vi "Replace Outside Typedef Const.vi"(8 "error in":errorcluster, 10 "non-library vi[]":string[](array[string]), 11 "target directory":path) -> (0 "error out":errorcluster)   [LabVIEW 2021, in "Converter.lvlib"]
uses:
  Converter.lvlib
  <vilib>/Utility/traverseref.llb/TRef TravTarget.ctl
  <vilib>/Utility/traverseref.llb/VI Scripting - Traverse.lvlib
  Converter Reusables/Converter Reusables.lvlib
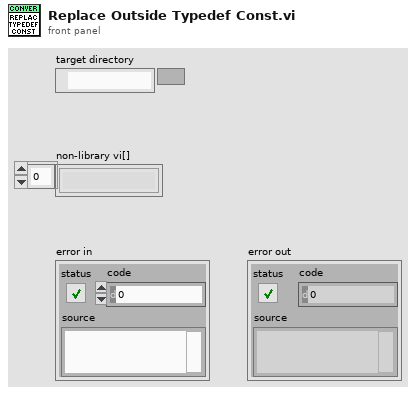
[diagram p1: front panel]
types:
  T1 = typedef "TRef TravTarget.ctl" = enum16{"FP", "BD", "Other"}
  T2 = enum32{"not a typedef", "typedef", "strict typedef", "class private data"}
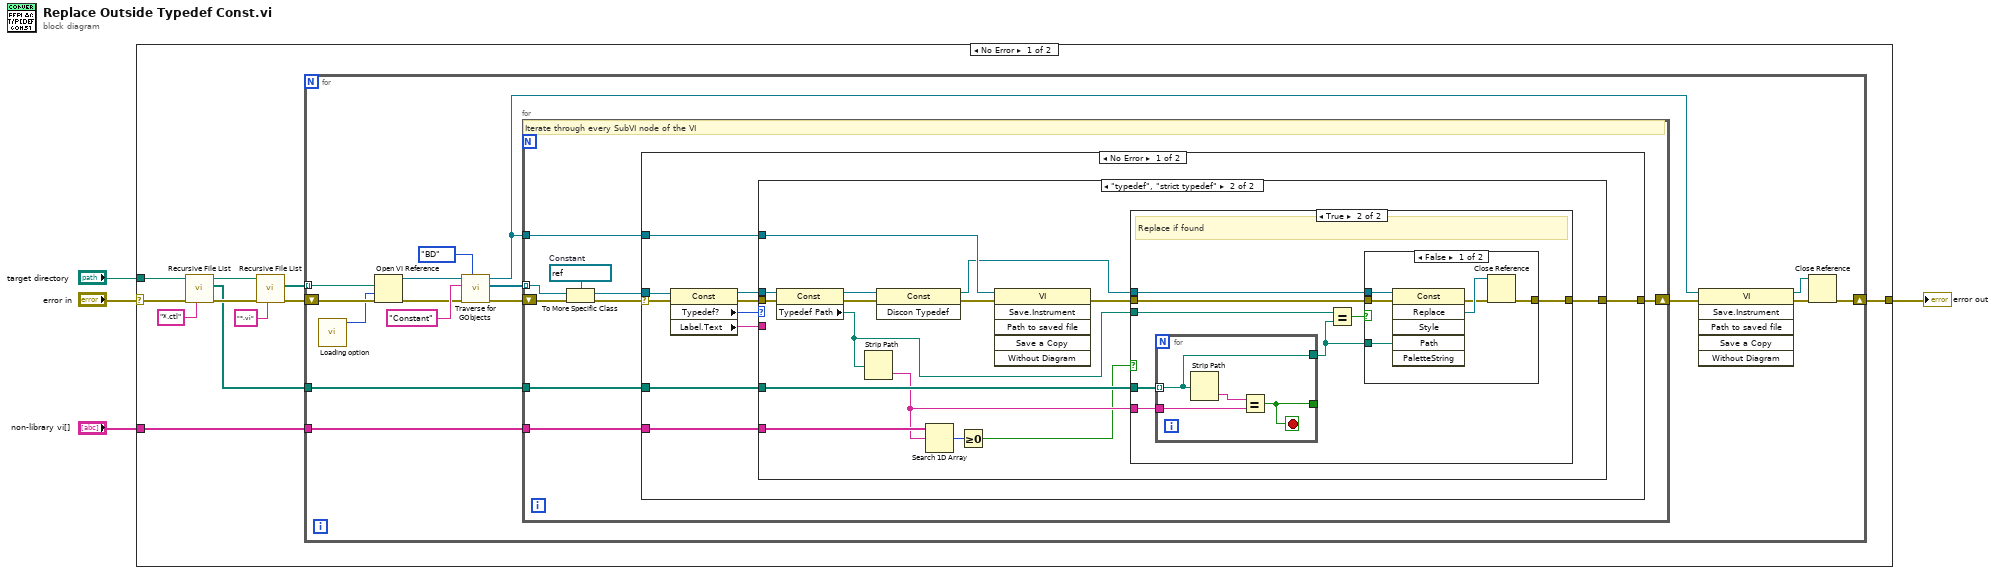
[diagram p0: block diagram]
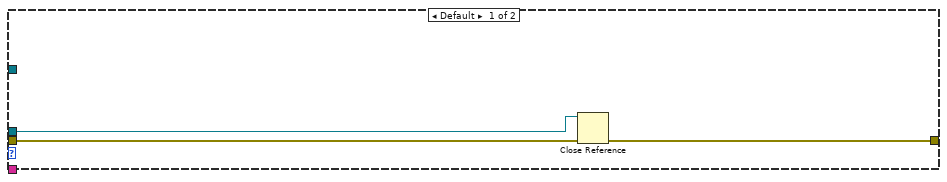
[diagram p2: hidden frame]
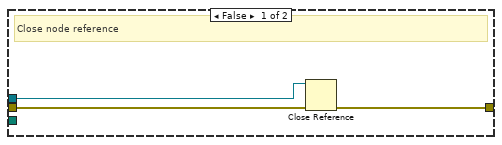
[diagram p3: hidden frame]
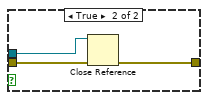
[diagram p4: hidden frame]
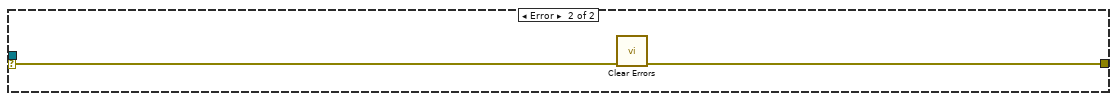
[diagram p5: hidden frame]
diagram:
  n1 = case shown="No Error" "error in" {
    selector: "error in" -> [w14 w95]
    tunnel: "non-library vi[]" -> [w15 _]
    tunnel: [w11 w95] -> w2
    tunnel: "target directory" -> [w9 _]
    frame No Error {
      n2 = call <vilib>:"Recursive File List.vi"("pattern"="*.ctl", "error in (no error)"=w14, "Folder Path"=w9) -> ("error out"=w10:errorcluster, "All Files in Dir"=w6:path[], "dup Folder Path"=w8:path)  [unwired: 4 in, 2 out]
      n3 = call <vilib>:"Recursive File List.vi"("pattern"="*.vi", "error in (no error)"=w10, "Folder Path"=w8) -> ("error out"=w13:errorcluster, "All Files in Dir"=w5:path[])  [unwired: 4 in, 3 out]
      n4 = for {
        tunnel: w6 -> [w30]
        tunnel: w15 -> [w29]
        tunnel: w5 -> [w21] mode=indexing
        shift-right: [w22] -> w11
        shift-left: w13 -> [w24]
        n5 = call "Loading option.vi"() -> ("options"=w16:i32)  [unwired: 11 in]
        n6 = Open VI Reference(vi path=w21, options=w16, error in (no error)=w24) -> (vi reference=w20:refnum<vi>, error out=w23:errorcluster)  [unwired: 3 in]
        n7 = call <vilib>:"Traverse for GObjects.vi"("Traverse Target"=TRef_TravTarget."BD", "error in (no error)"=w23, "Class Name"="Constant" ("name/order"), "VI Refnum"=w20) -> ("error out"=w28:errorcluster, "References"=w31:refnum<vi>[], "dup VI Refnum"=w17:refnum<vi>)  [unwired: 4 in, 1 out]
        n8 = for {
          tunnel: w31 -> [w40] mode=indexing
          shift-right: [w38] -> w27
          shift-left: w28 -> [w39]
          tunnel: w29 -> [w35]
          tunnel: w30 -> [w37]
          tunnel: w17 -> [w32]
          w36 = refnum<vi> refnum  # Constant
          # "Iterate through every SubVI node of the VI"
          n9 = To More Specific Class(target class=w36, reference=w40, error in=w39) -> (specific class reference=w33:refnum<vi>, error out=w34:errorcluster)
          n10 = case shown="No Error" w34 {
            selector: w34 -> [w43 w94]
            tunnel: [w48 w93] -> w38
            tunnel: w37 -> [w47 _]
            tunnel: w35 -> [w46 _]
            tunnel: w33 -> [w44 _]
            tunnel: w32 -> [w41 _]
            frame No Error {
              n11 = property class="Const"(reference=w44, error in=w43) -> (reference out=w49:refnum<vi>, error out=w50:errorcluster, "Typedef?"=w45:T2, "Label.Text"=w42:string)
              n12 = case shown="\"typedef\", \"strict typedef\"" w45 {
                tunnel: w50 -> [w53 w67]
                tunnel: w49 -> [w51 w63]
                tunnel: [w52 w66] -> w48
                tunnel: w47 -> [_ w65]
                tunnel: w46 -> [_ w64]
                tunnel: w42 -> [_ _]
                tunnel: w41 -> [_ w57]
                frame Default {
                  n13 = Close Reference(reference=w51, error in (no error)=w53) -> (error out=w52:errorcluster)
                }
                frame "typedef", "strict typedef" {
                  n14 = property class="Const"(reference=w63, error in=w67) -> (reference out=w61:refnum<vi>, error out=w60:errorcluster, "Typedef Path"=w54:path)
                  n15 = Strip Path(path=w54) -> (name=w62:string)  [unwired: 1 out]
                  n16 = invoke class="Const" method="Discon Typedef"(reference=w61, error in=w60) -> (reference out=w56:refnum<vi>, error out=w59:errorcluster)  [unwired: 1 in, 1 out]
                  n17 = Search 1D Array(1D array=w64, element=w62) -> (index of element=w68:i32)  [unwired: 1 in]
                  n18 = Greater Or Equal To 0?(x=w68) -> (x >= 0?=w55:bool)
                  n19 = invoke class="VI" method="Save.Instrument"(reference=w57, error in=w59) -> (error out=w58:errorcluster)  [unwired: 4 in, 5 out]
                  n20 = case shown="True" w55 {
                    tunnel: w58 -> [w71 w79]
                    tunnel: w56 -> [w70 w78]
                    tunnel: [w69 w75] -> w66
                    tunnel: w65 -> [_ w77]
                    tunnel: w62 -> [_ w76]
                    tunnel: w54 -> [_ w74]
                    frame False {
                      # "Close node reference"
                      n21 = Close Reference(reference=w70, error in (no error)=w71) -> (error out=w69:errorcluster)
                    }
                    frame True {
                      # "Replace if found"
                      n22 = for {
                        tunnel: w77 -> [w90] mode=indexing
                        tunnel: w76 -> [w91]
                        tunnel: [w90] -> w73
                        tunnel: [w89] -> _
                        stop <- w89 stop-if-true
                        n23 = Strip Path(path=w90) -> (name=w92:string)  [unwired: 1 out]
                        n24 = Equal?(x=w92, y=w91) -> (x = y?=w89:bool)
                      }
                      n25 = Equal?(x=w74, y=w73) -> (x = y?=w72:bool)
                      n26 = case shown="False" w72 {
                        tunnel: w79 -> [w85 w88]
                        tunnel: w78 -> [w84 w86]
                        tunnel: [w81 w87] -> w75
                        tunnel: w73 -> [w80 _]
                        frame False {
                          n27 = invoke class="Const" method="Replace"(reference=w84, error in=w85, "Path"=w80) -> (error out=w82:errorcluster, "Replace"=w83:refnum<vi>)  [unwired: 3 in, 4 out]
                          n28 = Close Reference(reference=w83, error in (no error)=w82) -> (error out=w81:errorcluster)
                        }
                        frame True {
                          n29 = Close Reference(reference=w86, error in (no error)=w88) -> (error out=w87:errorcluster)
                        }
                      }
                    }
                  }
                }
              }
            }
            frame Error {
              n30 = call <vilib>:"Clear Errors.vi"("error in (no error)"=w94) -> ("error out"=w93:errorcluster)  [unwired: 5 in, 1 out]
            }
          }
        }
        n31 = invoke class="VI" method="Save.Instrument"(reference=w17, error in=w27) -> (reference out=w18:refnum<vi>, error out=w19:errorcluster)  [unwired: 4 in, 4 out]
        n32 = Close Reference(reference=w18, error in (no error)=w19) -> (error out=w22:errorcluster)
      }
    }
    frame Error {
    }
  }
  "error out" <- w2
